vi "7 segmentos.vi"(8 "Numeric":u8) -> (0 "[6]":bool, 1 "[5]":bool, 2 "[4]":bool, 3 "[3]":bool, 4 "[2]":bool, 5 "[1]":bool, 6 "[0]":bool)   [LabVIEW 2020]
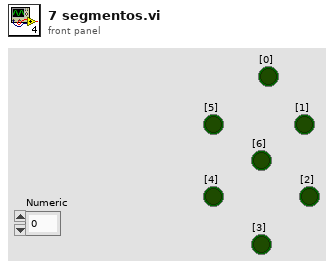
[diagram p1: front panel]
types:
  T1 = cluster{"[0]":bool, "[1]":bool, "[2]":bool, "[3]":bool, "[4]":bool, "[5]":bool, "[6]":bool, "[7]":bool, "[8]":bool}
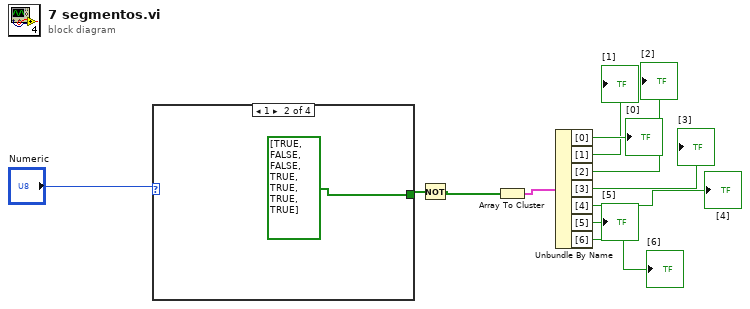
[diagram p0: block diagram]
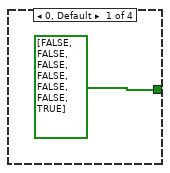
[diagram p2: hidden frame]
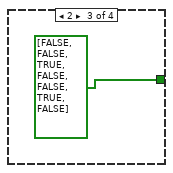
[diagram p3: hidden frame]
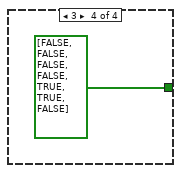
[diagram p4: hidden frame]
diagram:
  n1 = case shown="1" "Numeric" {
    tunnel: [bool[] [FALSE, FALSE, FALSE, FALSE, FALSE, FALSE, TRUE] bool[] [TRUE, FALSE, FALSE, TRUE, TRUE, TRUE, TRUE] bool[] [FALSE, FALSE, TRUE, FALSE, FALSE, TRUE, FALSE] bool[] [FALSE, FALSE, FALSE, FALSE, TRUE, TRUE, FALSE]] -> w8
    frame 0, Default {
    }
    frame 1 {
    }
    frame 2 {
    }
    frame 3 {
    }
  }
  n2 = Not(x=w8) -> (.not. x?=w9:bool[])
  n3 = Array To Cluster(array=w9) -> (cluster=w10:T1)
  n4 = Unbundle By Name(w10) -> ("[0]"=→"[0]":bool, "[1]"=→"[1]":bool, "[2]"=→"[2]":bool, "[3]"=→"[3]":bool, "[4]"=→"[4]":bool, "[5]"=→"[5]":bool, "[6]"=→"[6]":bool)
